vi "数据排序.vi"(7 "结果数字":string, 8 "总数":i32=11, 10 "原始数据":string[](array[string])) -> (3 "排序后结果输出":string[](array[string]), 4 "out":string[](array[string]))   [LabVIEW 2011]
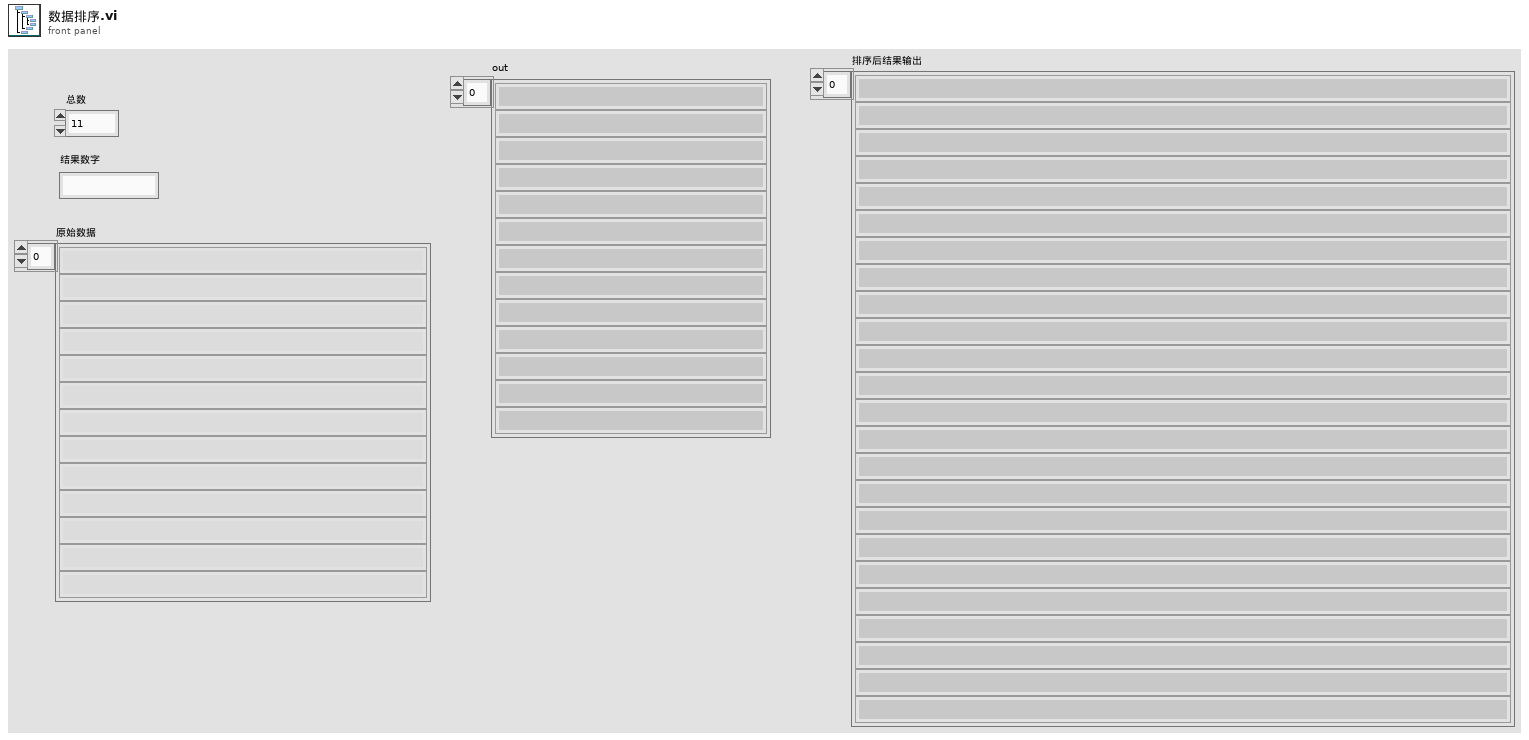
[diagram p1: front panel]
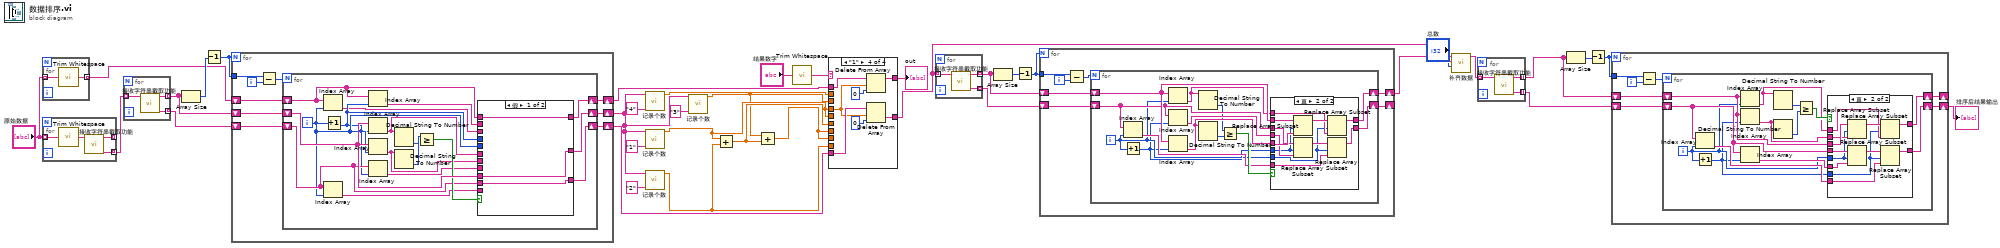
[diagram p0: block diagram]
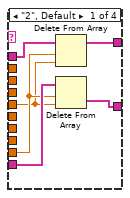
[diagram p4: hidden frame]
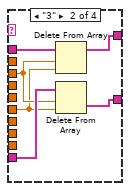
[diagram p5: hidden frame]
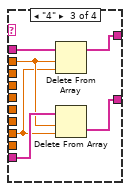
[diagram p6: hidden frame]
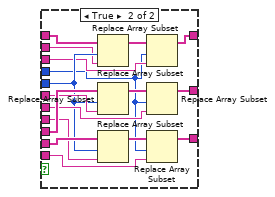
[diagram p7: hidden frame]
diagram:
  n1 = for {
    tunnel: "原始数据" -> [w38] mode=indexing
    tunnel: [w37] -> w10 mode=indexing
    n2 = call <vilib>:"Trim Whitespace.vi"("string"=w38) -> ("trimmed string"=w37:string)  [unwired: 1 in]
  }
  n3 = for {
    tunnel: "原始数据" -> [w40] mode=indexing
    tunnel: [w42] -> _ mode=indexing
    tunnel: [w41] -> w17 mode=indexing
    n4 = call <vilib>:"Trim Whitespace.vi"("string"=w40) -> ("trimmed string"=w39:string)  [unwired: 1 in]
    n5 = call "接收字符串截取功能.vi"("输入结果"=w39) -> ("输出结果"=w41:string, "工位名称"=w42:string)  [unwired: 9 in]
  }
  n6 = for {
    tunnel: w17 -> [w45] mode=indexing
    tunnel: [w44] -> w34 mode=indexing
    tunnel: [w43] -> w28 mode=indexing
    n7 = call "接收字符串截取功能.vi"("输入结果"=w45) -> ("输出结果"=w43:string, "工位名称"=w44:string)  [unwired: 9 in]
  }
  n8 = Array Size(array=w34) -> (size(s)=w36:i32)
  n9 = Decrement(x=w36) -> (x-1=w35:i32)
  n10 = for {
    N: w35 -> [_]
    shift-right: [w52] -> w30
    shift-left: w34 -> [w53]
    tunnel: w35 -> [w51]
    shift-right: [w48] -> w27
    shift-left: w28 -> [w54]
    shift-right: [w46] -> w26
    shift-left: w10 -> [w47]
    i -> [w50]
    n11 = Subtract(x=w51, y=w50) -> (x-y=w49:i32)
    n12 = for {
      N: w49 -> [_]
      shift-right: [w70] -> w52
      shift-left: w53 -> [w71]
      shift-right: [w68] -> w48
      shift-left: w54 -> [w67]
      shift-right: [w59] -> w46
      shift-left: w47 -> [w64]
      i -> [w63]
      n13 = Index Array(array=w64, index=w63) -> (element=w61:string)
      n14 = Index Array(array=w67, index=w63) -> (element=w66:string)
      n15 = Increment(x=w63) -> (x+1=w62:i32)
      n16 = Index Array(array=w64, index=w62) -> (element=w60:string)
      n17 = Index Array(array=w71, index=w62) -> (element=w57:string)
      n18 = Index Array(array=w71, index=w63) -> (element=w58:string)
      n19 = Index Array(array=w67, index=w62) -> (element=w65:string)
      n20 = Decimal String To Number(string=w57) -> (number=w55:i32)  [unwired: 2 in, 1 out]
      n21 = Decimal String To Number(string=w58) -> (number=w56:i32)  [unwired: 2 in, 1 out]
      n22 = Greater Or Equal?(x=w56, y=w55) -> (x >= y?=w69:bool)
      n23 = case shown="假" w69 {
        tunnel: w63 -> [_ w80]
        tunnel: w71 -> [w74 w91]
        tunnel: w62 -> [_ w77]
        tunnel: w57 -> [_ w90]
        tunnel: w58 -> [_ w88]
        tunnel: [w74 w87] -> w70
        tunnel: w67 -> [w73 w86]
        tunnel: [w73 w84] -> w68
        tunnel: w66 -> [_ w82]
        tunnel: w65 -> [_ w83]
        tunnel: w64 -> [w72 w81]
        tunnel: w61 -> [_ w79]
        tunnel: w60 -> [_ w78]
        tunnel: [w72 w75] -> w59
        frame False {
        }
        frame True {
          n24 = Replace Array Subset(array=w81, new element=w78, index=w80) -> (w76:string[])
          n25 = Replace Array Subset(array=w91, new element=w90, index=w80) -> (w89:string[])
          n26 = Replace Array Subset(array=w86, new element=w83, index=w80) -> (w85:string[])
          n27 = Replace Array Subset(array=w76, new element=w79, index=w77) -> (w75:string[])
          n28 = Replace Array Subset(array=w89, new element=w88, index=w77) -> (w87:string[])
          n29 = Replace Array Subset(array=w85, new element=w82, index=w77) -> (w84:string[])
        }
      }
    }
  }
  n30 = call "记录个数.vi"("索引字符串"="4", "原始数据输入"=w30) -> ("结果个数输出"=w23:dbl)  [unwired: 9 in]
  n31 = call "记录个数.vi"("索引字符串"="1", "原始数据输入"=w30) -> ("结果个数输出"=w25:dbl)  [unwired: 9 in]
  n32 = call "记录个数.vi"("索引字符串"="2", "原始数据输入"=w30) -> ("结果个数输出"=w15:dbl)  [unwired: 9 in]
  n33 = call "记录个数.vi"("索引字符串"="3", "原始数据输入"=w30) -> ("结果个数输出"=w14:dbl)  [unwired: 9 in]
  n34 = Add(x=w25, y=w15) -> (x+y=w24:dbl)
  n35 = Add(x=w14, y=w24) -> (x+y=w22:dbl)
  n36 = call <vilib>:"Trim Whitespace.vi"("string"="结果数字") -> ("trimmed string"=w12:string)  [unwired: 1 in]
  n37 = case shown="\"1\"" w12 {
    tunnel: w22 -> [_ _ _ _]
    tunnel: w27 -> [w97 w103 w109 w116]
    tunnel: w26 -> [w95 w102 w108 w112]
    tunnel: w25 -> [_ _ _ w111]
    tunnel: [w96 w99 w104 w114] -> w8
    tunnel: [w94 w98 w105 w110] -> w16
    tunnel: w25 -> [w92 _ _ _]
    tunnel: w15 -> [w93 _ _ _]
    tunnel: w14 -> [_ w101 _ _]
    tunnel: w24 -> [_ w100 _ _]
    tunnel: w23 -> [_ _ w107 _]
    tunnel: w22 -> [_ _ w106 _]
    frame "2", Default {
      n38 = Delete From Array(array=w95, length=w93, index=w92) -> (array with subset deleted=w94:string[])  [unwired: 1 out]
      n39 = Delete From Array(array=w97, length=w93, index=w92) -> (deleted portion=w96:string[])  [unwired: 1 out]
    }
    frame "3" {
      n40 = Delete From Array(array=w102, length=w101, index=w100) -> (array with subset deleted=w98:string[])  [unwired: 1 out]
      n41 = Delete From Array(array=w103, length=w101, index=w100) -> (deleted portion=w99:string[])  [unwired: 1 out]
    }
    frame "4" {
      n42 = Delete From Array(array=w108, length=w107, index=w106) -> (array with subset deleted=w105:string[])  [unwired: 1 out]
      n43 = Delete From Array(array=w109, length=w107, index=w106) -> (deleted portion=w104:string[])  [unwired: 1 out]
    }
    frame "1" {
      n44 = Delete From Array(array=w112, length=w111, index=0 ("索引")) -> (array with subset deleted=w110:string[])  [unwired: 1 out]
      n45 = Delete From Array(array=w116, length=w111, index=0 ("索引")) -> (deleted portion=w114:string[])  [unwired: 1 out]
    }
  }
  "out" <- w16
  n46 = for {
    tunnel: w8 -> [w119] mode=indexing
    tunnel: [w118] -> w19 mode=indexing
    tunnel: [w117] -> w18 mode=indexing
    n47 = call "接收字符串截取功能.vi"("输入结果"=w119) -> ("输出结果"=w117:string, "工位名称"=w118:string)  [unwired: 9 in]
  }
  n48 = Array Size(array=w19) -> (size(s)=w21:i32)
  n49 = Decrement(x=w21) -> (x-1=w20:i32)
  n50 = for {
    N: w20 -> [_]
    shift-right: [w124] -> w9
    shift-left: w19 -> [w125]
    tunnel: w20 -> [w123]
    shift-right: [w120] -> _
    shift-left: w18 -> [w126]
    i -> [w122]
    n51 = Subtract(x=w123, y=w122) -> (x-y=w121:i32)
    n52 = for {
      N: w121 -> [_]
      shift-right: [w138] -> w124
      shift-left: w125 -> [w139]
      shift-right: [w136] -> w120
      shift-left: w126 -> [w135]
      i -> [w132]
      n53 = Index Array(array=w135, index=w132) -> (element=w134:string)
      n54 = Increment(x=w132) -> (x+1=w131:i32)
      n55 = Index Array(array=w139, index=w132) -> (element=w129:string)
      n56 = Index Array(array=w135, index=w131) -> (element=w133:string)
      n57 = Index Array(array=w139, index=w131) -> (element=w130:string)
      n58 = Decimal String To Number(string=w129) -> (number=w128:i32)  [unwired: 2 in, 1 out]
      n59 = Decimal String To Number(string=w130) -> (number=w127:i32)  [unwired: 2 in, 1 out]
      n60 = Greater Or Equal?(x=w128, y=w127) -> (x >= y?=w137:bool)
      n61 = case shown="真" w137 {
        tunnel: w132 -> [_ w143]
        tunnel: w139 -> [w141 w153]
        tunnel: w131 -> [_ w142]
        tunnel: w130 -> [_ w152]
        tunnel: w129 -> [_ w150]
        tunnel: [w141 w149] -> w138
        tunnel: w135 -> [w140 w148]
        tunnel: [w140 w146] -> w136
        tunnel: w134 -> [_ w144]
        tunnel: w133 -> [_ w145]
        frame False {
        }
        frame True {
          n62 = Replace Array Subset(array=w153, new element=w152, index=w143) -> (w151:string[])
          n63 = Replace Array Subset(array=w148, new element=w145, index=w143) -> (w147:string[])
          n64 = Replace Array Subset(array=w151, new element=w150, index=w142) -> (w149:string[])
          n65 = Replace Array Subset(array=w147, new element=w144, index=w142) -> (w146:string[])
        }
      }
    }
  }
  n66 = call "补齐数据.vi"("总数"="总数", "排序后结果输入"=w8, "數字"=w9) -> ("排序后结果输出"=w2:string[])  [unwired: 8 in]
  n67 = for {
    tunnel: w2 -> [w156] mode=indexing
    tunnel: [w155] -> w5 mode=indexing
    tunnel: [w154] -> w6 mode=indexing
    n68 = call "接收字符串截取功能.vi"("输入结果"=w156) -> ("输出结果"=w154:string, "工位名称"=w155:string)  [unwired: 9 in]
  }
  n69 = Array Size(array=w5) -> (size(s)=w3:i32)
  n70 = Decrement(x=w3) -> (x-1=w4:i32)
  n71 = for {
    N: w4 -> [_]
    shift-right: [w161] -> _
    shift-left: w5 -> [w162]
    tunnel: w4 -> [w160]
    shift-right: [w157] -> w1
    shift-left: w6 -> [w163]
    i -> [w159]
    n72 = Subtract(x=w160, y=w159) -> (x-y=w158:i32)
    n73 = for {
      N: w158 -> [_]
      shift-right: [w175] -> w161
      shift-left: w162 -> [w176]
      shift-right: [w173] -> w157
      shift-left: w163 -> [w172]
      i -> [w169]
      n74 = Index Array(array=w172, index=w169) -> (element=w171:string)
      n75 = Increment(x=w169) -> (x+1=w168:i32)
      n76 = Index Array(array=w176, index=w169) -> (element=w165:string)
      n77 = Index Array(array=w176, index=w168) -> (element=w167:string)
      n78 = Index Array(array=w172, index=w168) -> (element=w170:string)
      n79 = Decimal String To Number(string=w165) -> (number=w164:i32)  [unwired: 2 in, 1 out]
      n80 = Decimal String To Number(string=w167) -> (number=w166:i32)  [unwired: 2 in, 1 out]
      n81 = Greater Or Equal?(x=w164, y=w166) -> (x >= y?=w174:bool)
      n82 = case shown="真" w174 {
        tunnel: w169 -> [_ w180]
        tunnel: w176 -> [w178 w190]
        tunnel: w168 -> [_ w179]
        tunnel: w167 -> [_ w189]
        tunnel: w165 -> [_ w187]
        tunnel: [w178 w186] -> w175
        tunnel: w172 -> [w177 w185]
        tunnel: [w177 w183] -> w173
        tunnel: w171 -> [_ w181]
        tunnel: w170 -> [_ w182]
        frame False {
        }
        frame True {
          n83 = Replace Array Subset(array=w190, new element=w189, index=w180) -> (w188:string[])
          n84 = Replace Array Subset(array=w185, new element=w182, index=w180) -> (w184:string[])
          n85 = Replace Array Subset(array=w188, new element=w187, index=w179) -> (w186:string[])
          n86 = Replace Array Subset(array=w184, new element=w181, index=w179) -> (w183:string[])
        }
      }
    }
  }
  "排序后结果输出" <- w1
